vi "String To Indexed Enum.vi"(7 "Variant":variant, 8 "error in (no error)":errorcluster, 11 "String":string) -> (0 "error out":errorcluster, 3 "Enum":variant)   [LabVIEW 2017]
doc: "Converts a string into an enum value, either from a leading index number or by matching the string against the enum labels case-insensitively."
uses:
  _openG/_reuse_openG.lvlib
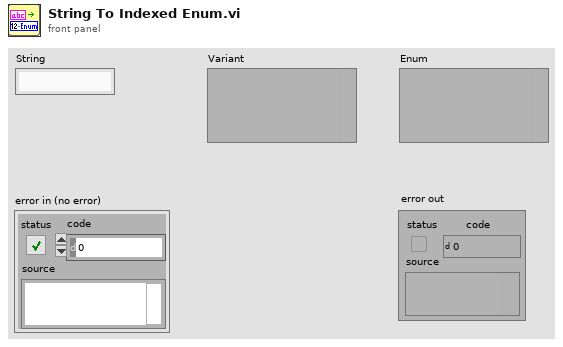
[diagram p1: front panel]
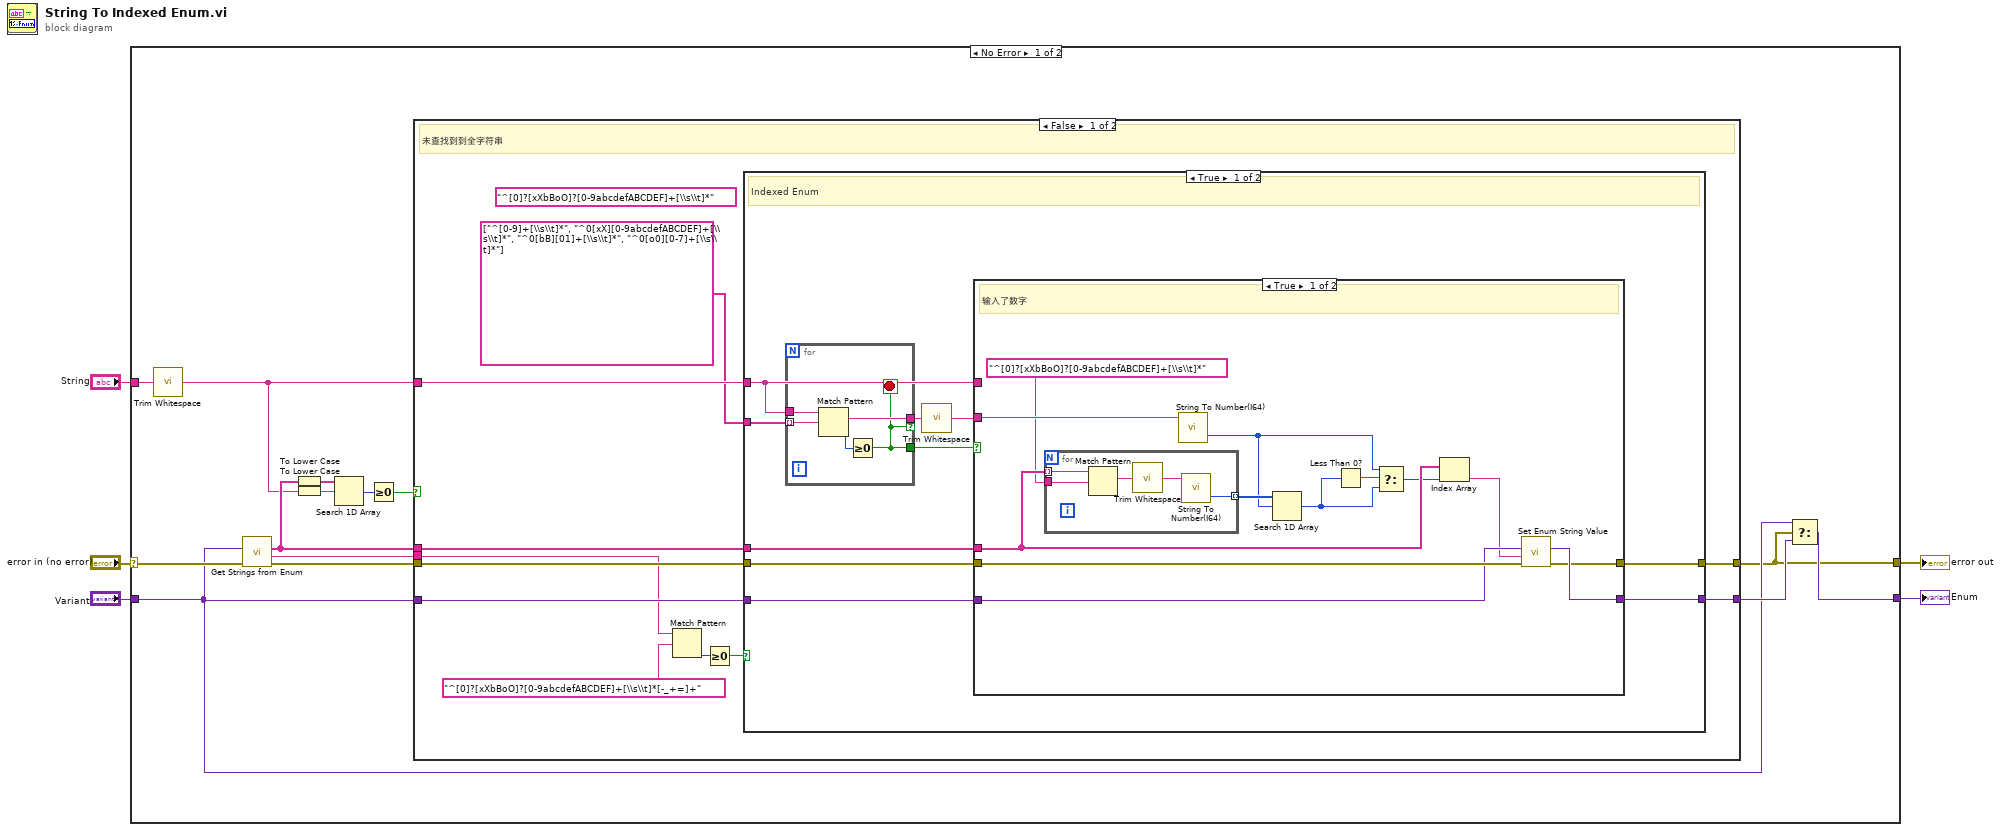
[diagram p0: block diagram]
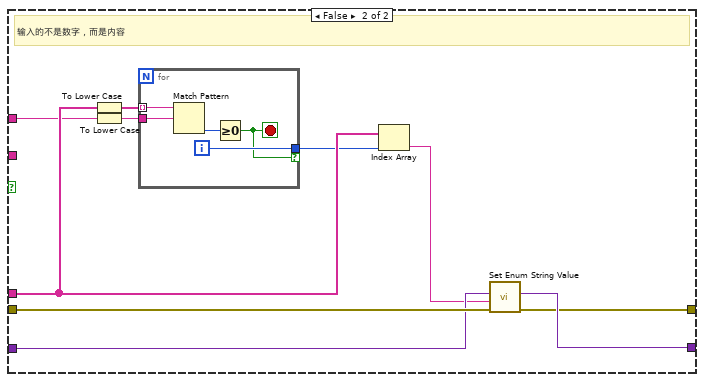
[diagram p2: hidden frame]
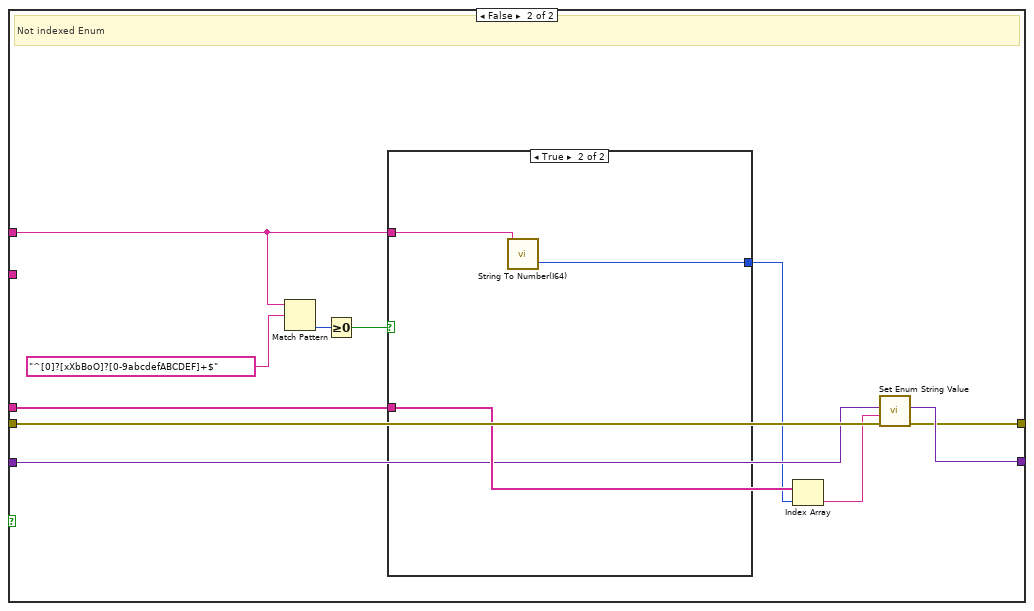
[diagram p3: hidden frame]
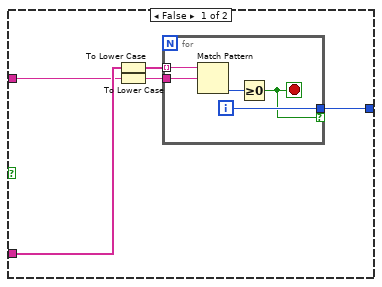
[diagram p4: hidden frame]
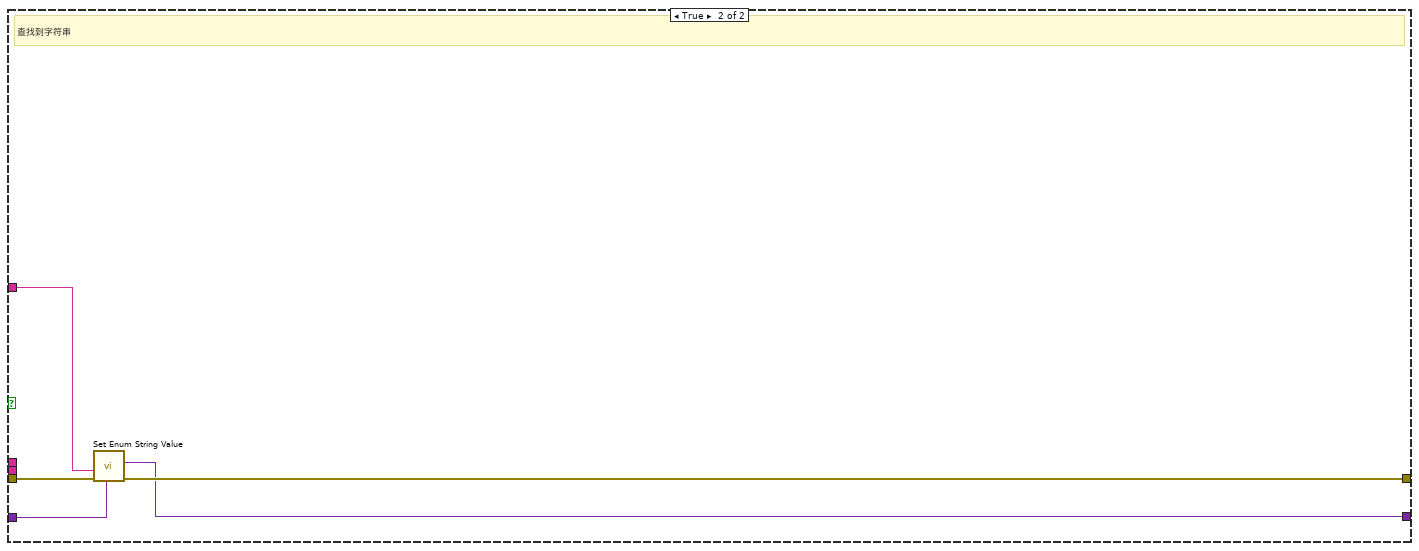
[diagram p5: hidden frame]
diagram:
  n1 = case shown="No Error" "error in (no error)" {
    selector: "error in (no error)" -> [w19 w108]
    tunnel: "Variant" -> [w15 w107]
    tunnel: "String" -> [w17 _]
    tunnel: [w14 w107] -> w2
    tunnel: [w13 w108] -> w1
    frame No Error {
      n2 = call <vilib>:"Trim Whitespace.vi"("string"=w17) -> ("trimmed string"=w7:string)  [unwired: 1 in]
      n3 = call "Get Strings from Enum.vi"("error in (no error)"=w19, "Enum"=w15) -> ("error out"=w18:errorcluster, "String Value"=w12:string, "Enum Strings"=w8:string[])  [unwired: 6 in, 1 out]
      n4 = To Lower Case(string=w8) -> (all lower case string=w9:string[])
      n5 = To Lower Case(string=w7) -> (all lower case string=w10:string)
      n6 = Search 1D Array(1D array=w9, element=w10) -> (index of element=w11:i32)  [unwired: 1 in]
      n7 = Greater Or Equal To 0?(x=w11) -> (x >= 0?=w6:bool)
      n8 = case shown="False" w6 {
        tunnel: w18 -> [w30 w106]
        tunnel: [w29 w102] -> w16
        tunnel: w15 -> [w28 w105]
        tunnel: [w27 w103] -> w13
        tunnel: w12 -> [w25 _]
        tunnel: w8 -> [w22 _]
        tunnel: w7 -> [w21 w104]
        frame False {
          (unwired) "^[0]?[xXbBoO]?[0-9abcdefABCDEF]+[\\s\\t]*" ("regular expression")
          # "未查找到到全字符串"
          n9 = Match Pattern(string=w25, regular expression="^[0]?[xXbBoO]?[0-9abcdefABCDEF]+[\\s\\t]*[-_+=]+") -> (offset past match=w26:i32)  [unwired: 1 in, 3 out]
          n10 = Greater Or Equal To 0?(x=w26) -> (x >= 0?=w23:bool)
          n11 = case shown="True" w23 {
            tunnel: w30 -> [w40 w89]
            tunnel: w22 -> [w36 w88]
            tunnel: w21 -> [w33 w81]
            tunnel: [w39 w87] -> w29
            tunnel: w28 -> [w38 w86]
            tunnel: [w37 w85] -> w27
            tunnel: string[] ["^[0-9]+[\\s\\t]*", "^0[xX][0-9abcdefABCDEF]+[\\s\\t]*", "^0[bB][01]+[\\s\\t]*", "^0[o0][0-7]+[\\s\\t]*"] -> [w32 _]
            frame True {
              # "Indexed Enum"
              n12 = for {
                tunnel: w32 -> [w41] mode=indexing
                tunnel: w33 -> [w45]
                tunnel: [w44] -> w35 if=w42
                tunnel: [w42] -> w31
                stop <- w42 stop-if-true
                n13 = Match Pattern(string=w45, regular expression=w41) -> (match substring=w44:string, offset past match=w43:i32)  [unwired: 1 in, 2 out]
                n14 = Greater Or Equal To 0?(x=w43) -> (x >= 0?=w42:bool)
              }
              n15 = call <vilib>:"Trim Whitespace.vi"("string"=w35) -> ("trimmed string"=w34:string)  [unwired: 1 in]
              n16 = case shown="True" w31 {
                tunnel: [w58 w73] -> w39
                tunnel: w40 -> [w57 w72]
                tunnel: w38 -> [w56 w71]
                tunnel: [w55 w70] -> w37
                tunnel: w36 -> [w54 w69]
                tunnel: w33 -> [_ w66]
                tunnel: w34 -> [w53 _]
                frame True {
                  # "输入了数字"
                  n17 = for {
                    tunnel: w54 -> [w63] mode=indexing
                    tunnel: [w59] -> w51 mode=indexing
                    tunnel: "^[0]?[xXbBoO]?[0-9abcdefABCDEF]+[\\s\\t]*" ("regular expression") -> [w62]
                    n18 = Match Pattern(string=w63, regular expression=w62) -> (match substring=w61:string)  [unwired: 1 in, 3 out]
                    n19 = call <vilib>:"Trim Whitespace.vi"("string"=w61) -> ("trimmed string"=w60:string)  [unwired: 1 in]
                    n20 = call "String To Number(I64).vi"("String"=w60) -> ("Numeric(I64)"=w59:i64)  [unwired: 4 in]
                  }
                  n21 = call "String To Number(I64).vi"("String"=w53) -> ("Numeric(I64)"=w48:i64)  [unwired: 4 in]
                  n22 = Search 1D Array(1D array=w51, element=w48) -> (index of element=w49:i32)  [unwired: 1 in]
                  n23 = Less Than 0?(x=w49) -> (x < 0?=w50:bool)
                  n24 = Select(t=w48, s=w50, f=w49) -> (s? t:f=w47:i64)
                  n25 = Index Array(array=w54, index=w47) -> (element=w52:string)
                  n26 = call "Set Enum String Value.vi"("error in (no error)"=w57, "String Value"=w52, "Default Enum Value"=w56) -> ("error out"=w55:errorcluster, "Enum"=w58:variant)  [unwired: 7 in]
                }
                frame False {
                  # "输入的不是数字，而是内容"
                  n27 = To Lower Case(string=w69) -> (all lower case string=w65:string[])
                  n28 = To Lower Case(string=w66) -> (all lower case string=w64:string)
                  n29 = for {
                    tunnel: w65 -> [w78] mode=indexing
                    tunnel: w64 -> [w77]
                    tunnel: [w76] -> w68 if=w74
                    i -> [w76]
                    stop <- w74 stop-if-true
                    n30 = Match Pattern(string=w78, regular expression=w77) -> (offset past match=w75:i32)  [unwired: 1 in, 3 out]
                    n31 = Greater Or Equal To 0?(x=w75) -> (x >= 0?=w74:bool)
                  }
                  n32 = Index Array(array=w69, index=w68) -> (element=w67:string)
                  n33 = call "Set Enum String Value.vi"("error in (no error)"=w72, "String Value"=w67, "Default Enum Value"=w71) -> ("error out"=w70:errorcluster, "Enum"=w73:variant)  [unwired: 7 in]
                }
              }
            }
            frame False {
              # "Not indexed Enum"
              n34 = Match Pattern(string=w81, regular expression="^[0]?[xXbBoO]?[0-9abcdefABCDEF]+$") -> (offset past match=w80:i32)  [unwired: 1 in, 3 out]
              n35 = Greater Or Equal To 0?(x=w80) -> (x >= 0?=w79:bool)
              n36 = case shown="True" w79 {
                tunnel: w88 -> [w94 _]
                tunnel: [w93 w100] -> w84
                tunnel: w81 -> [w90 w101]
                frame False {
                  n37 = To Lower Case(string=w94) -> (all lower case string=w92:string[])
                  n38 = To Lower Case(string=w90) -> (all lower case string=w91:string)
                  n39 = for {
                    tunnel: w92 -> [w99] mode=indexing
                    tunnel: w91 -> [w98]
                    tunnel: [w97] -> w93 if=w95
                    i -> [w97]
                    stop <- w95 stop-if-true
                    n40 = Match Pattern(string=w99, regular expression=w98) -> (offset past match=w96:i32)  [unwired: 1 in, 3 out]
                    n41 = Greater Or Equal To 0?(x=w96) -> (x >= 0?=w95:bool)
                  }
                }
                frame True {
                  n42 = call "String To Number(I64).vi"("String"=w101) -> ("Numeric(I64)"=w100:i64)  [unwired: 4 in]
                }
              }
              n43 = Index Array(array=w88, index=w84) -> (element=w83:string)
              n44 = call "Set Enum String Value.vi"("error in (no error)"=w89, "String Value"=w83, "Default Enum Value"=w86) -> ("error out"=w85:errorcluster, "Enum"=w87:variant)  [unwired: 7 in]
            }
          }
        }
        frame True {
          # "查找到字符串"
          n45 = call "Set Enum String Value.vi"("error in (no error)"=w106, "String Value"=w104, "Default Enum Value"=w105) -> ("error out"=w103:errorcluster, "Enum"=w102:variant)  [unwired: 7 in]
        }
      }
      n46 = Select(t=w15, s=w13, f=w16) -> (s? t:f=w14:variant)
    }
    frame Error {
    }
  }
  "Enum" <- w2
  "error out" <- w1
